vi "Wrist Control.vi"(6 "Case for Wrist":dbl, 8 "Arm Position":dbl, 9 "Position offset":dbl, 10 "Manual Wrist move":dbl format="%#_13g", 11 "Wrist Position":dbl) -> (2 "Wrist Position":dbl, 3 "Position offset":dbl)   [LabVIEW 2014]
uses:
  Robot Global Data.vi
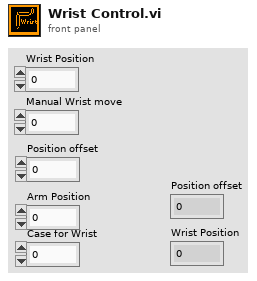
[diagram p1: front panel]
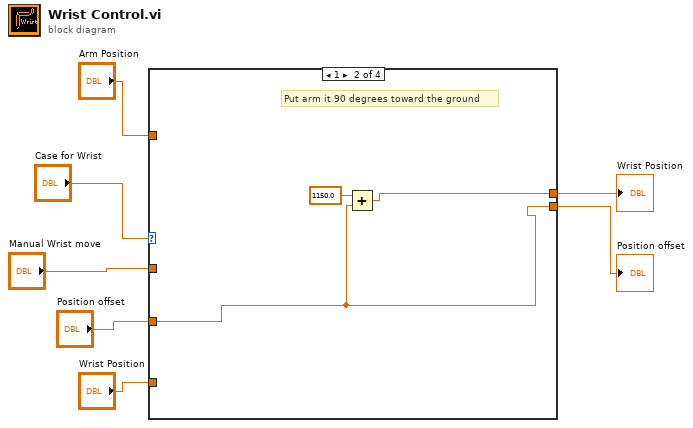
[diagram p0: block diagram]
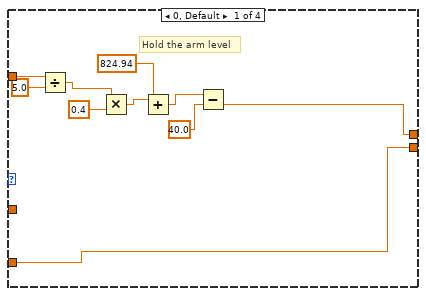
[diagram p2: hidden frame]
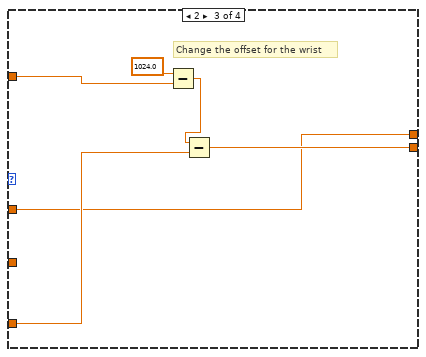
[diagram p3: hidden frame]
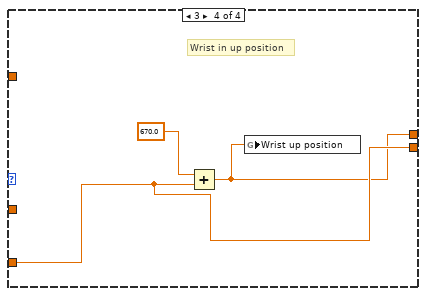
[diagram p4: hidden frame]
diagram:
  n1 = case shown="1" "Case for Wrist" {
    tunnel: "Arm Position" -> [w10 _ w26 _]
    tunnel: "Position offset" -> [w17 w19 _ w29]
    tunnel: [w13 w20 w21 w27] -> w4
    tunnel: "Wrist Position" -> [_ _ w23 _]
    tunnel: [w17 w19 w22 w29] -> w2
    tunnel: "Manual Wrist move" -> [_ _ w21 _]
    frame 0, Default {
      # "Hold the arm level"
      n2 = Divide(x=w10, y=5.0) -> (x/y=w8:dbl)
      n3 = Multiply(x=w8, y=0.4) -> (x*y=w15:dbl)
      n4 = Add(x=w15, y=824.94) -> (x+y=w12:dbl)
      n5 = Subtract(x=w12, y=40.0) -> (x-y=w13:dbl)
    }
    frame 1 {
      # "Put arm it 90 degrees toward the ground"
      n6 = Add(x=1150.0, y=w19) -> (x+y=w20:dbl)
    }
    frame 2 {
      # "Change the offset for the wrist"
      n7 = Subtract(x=1024.0, y=w26) -> (x-y=w24:dbl)
      n8 = Subtract(x=w24, y=w23) -> (x-y=w22:dbl)
    }
    frame 3 {
      # "Wrist in up position"
      n9 = Add(x=670.0, y=w29) -> (x+y=w27:dbl)
      n10 = global write "Robot Global Data.vi" "Wrist up position"(w27) -> ()
    }
  }
  "Wrist Position" <- w4
  "Position offset" <- w2
